vi "10_3.vi"() -> ()   [LabVIEW 2026]
panel:
  out "set 2":set{dbl[]}(c389)
  in  "element":dbl
  in  "Numeric 2":dbl
  out "set":set{dbl}(c389)
  in  "Numeric":dbl
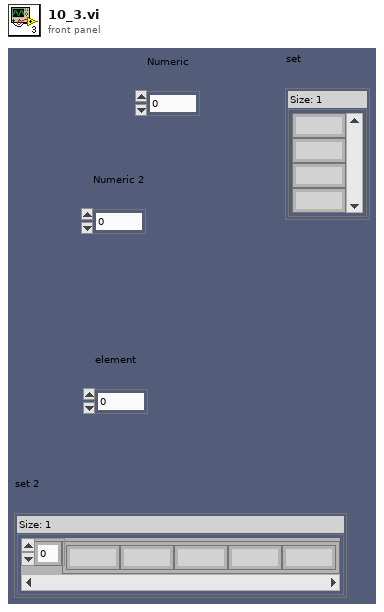
[diagram p1: front panel]
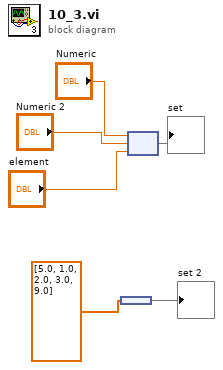
[diagram p0: block diagram]
diagram:
  n1 = node(dbl[] [5.0, 1.0, 2.0, 3.0, 9.0]) -> (→"set 2":set{dbl[]})
  n2 = node("Numeric", "Numeric 2", "element") -> (→"set":set{dbl})
